vi "NBreset.vi"(4 "Controller Device Description":string="DLP-IO20") -> ()   [LabVIEW 2013]
uses:
  Global 1.vi
panel:
  out "OK":bool
  out "Ping result":u8 format="%x"
  out "Status":i32=1
  out "Bytes Written 6":i32=5
  out "Bytes Read 6":i32
  out "Read Array 6":i32[](array[numeric])
  out "Write Array 6":i32[](array[numeric])=[5, 53, 6, 0, 0]
  out "Bytes Written 7":i32=5
  out "Bytes Read 7":i32
  out "Read Array 7":i32[](array[numeric])
  out "Write Array 7":i32[](array[numeric])=[5, 53, 7, 0, 0]
  out "Handle":u32=263961288
  # "Netburner Reset Panel"
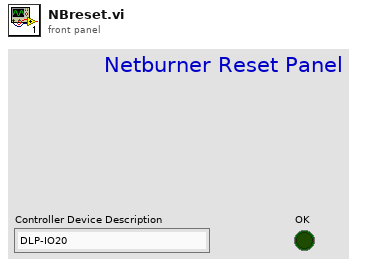
[diagram p1: front panel]
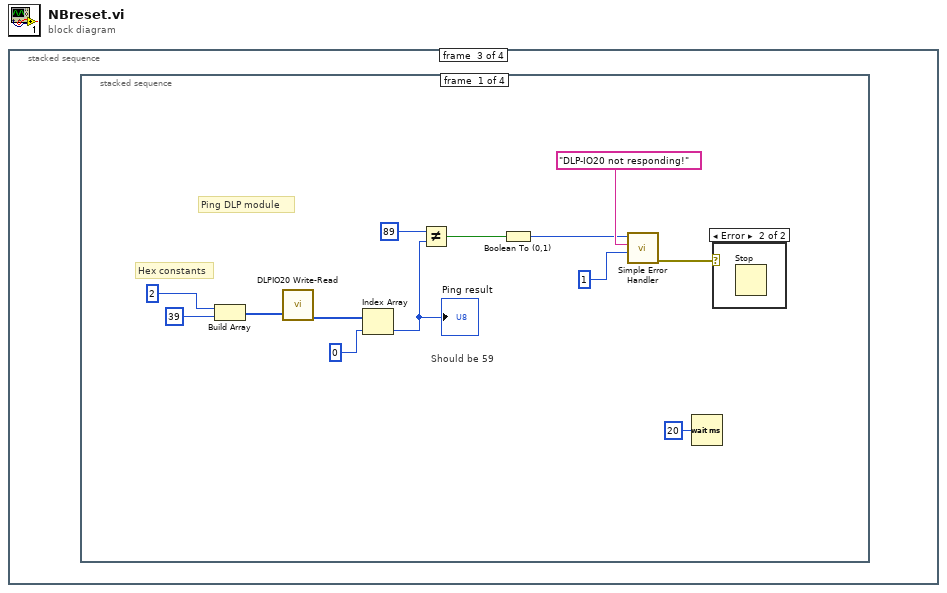
[diagram p0: block diagram]
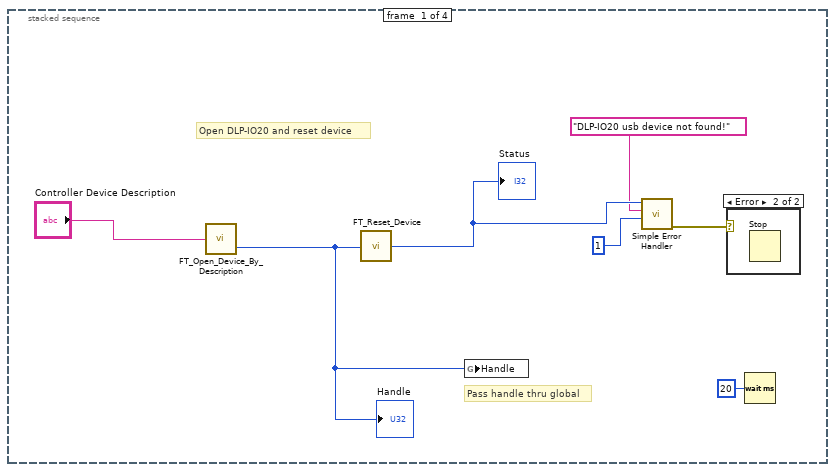
[diagram p2: hidden frame]
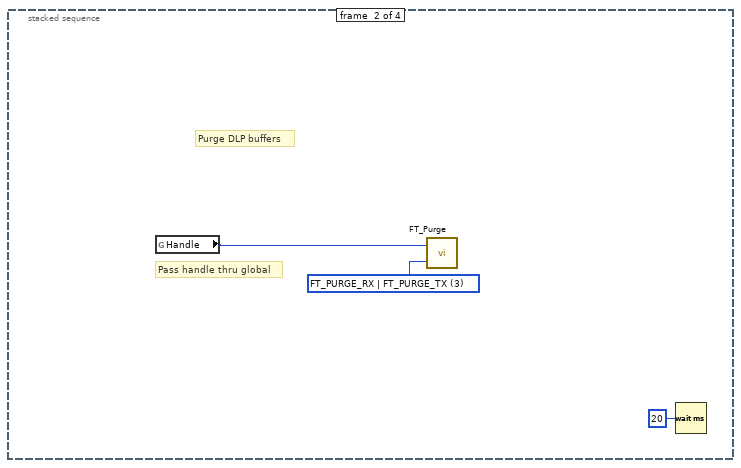
[diagram p4: hidden frame]
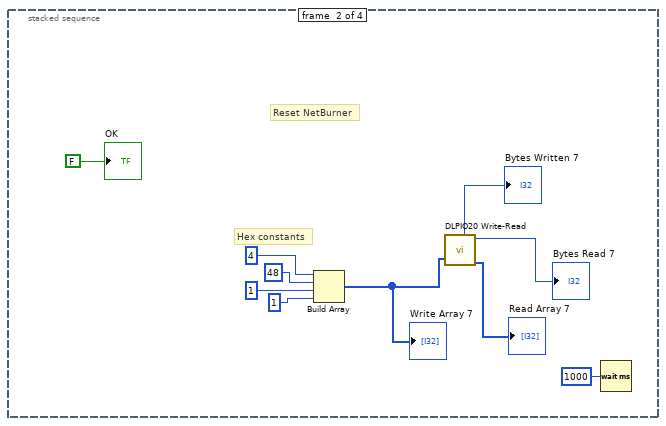
[diagram p6: hidden frame]
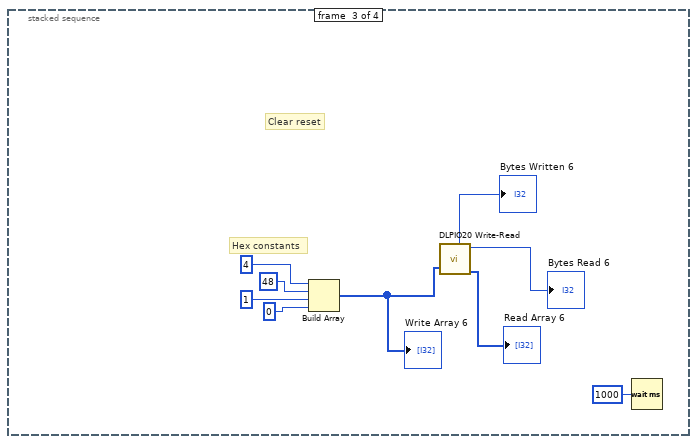
[diagram p7: hidden frame]
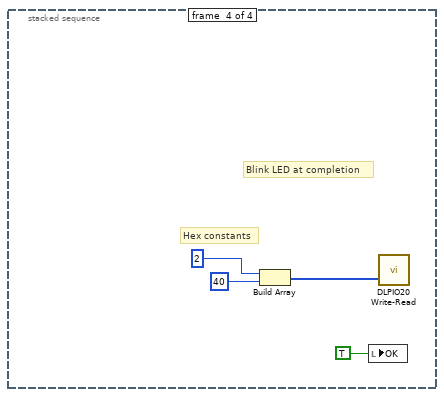
[diagram p8: hidden frame]
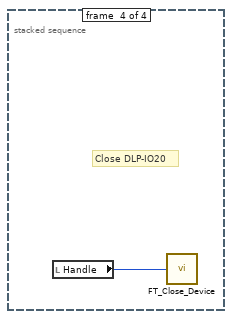
[diagram p9: hidden frame]
diagram:
  n1 = stacked-sequence {
    frame #0 {
      # "Pass handle thru global"
      # "Open DLP-IO20 and reset device"
      n2 = call "FT_Open_Device_By_Description.vi"("Device Description"="Controller Device Description") -> ("Handle"=w5:u32)  [unwired: 1 out]
      "Handle" <- w5
      n3 = call "FT_Reset_Device.vi"("Handle"=w5) -> ("FT_Status"=w4:u32)
      "Status" <- w4
      n4 = global write "Global 1.vi" "Handle"(w5) -> ()
      n5 = call <vilib>:"Simple Error Handler.vi"("error code (no error:0)"=w4, "error source (\" \")"="DLP-IO20 usb device not found!", "type of dialog (OK msg:1)"=1) -> ("error out"=w1:errorcluster)  [unwired: 2 in, 4 out]
      n6 = case shown="Error" w1 {
        frame No Error {
        }
        frame Error {
          n7 = Stop() -> ()  [unwired: 1 in]
        }
      }
      n8 = Wait (ms)(milliseconds to wait=u32 20) -> ()  [unwired: 1 out]
    }
    frame #1 {
      w10 = u32 3 items=["FT_PURGE_RX"=1, "FT_PURGE_TX"=2, "FT_PURGE_RX | FT_PURGE_TX"=3] ("Purge Flags")
      # "Purge DLP buffers"
      # "Pass handle thru global"
      n9 = global read "Global 1.vi" "Handle"() -> (w9:u32)
      n10 = call "FT_Purge.vi"("Purge Flags"=w10, "Handle"=w9) -> ()  [unwired: 1 out]
      n11 = Wait (ms)(milliseconds to wait=u32 20) -> ()  [unwired: 1 out]
    }
    frame #2 {
      n12 = stacked-sequence {
        frame #0 {
          # "Should be 59"
          # "Ping DLP module"
          # "Hex constants"
          n13 = Build Array "Build Array"(u8 2, u8 39) -> (w21:u8[])
          n14 = call "DLPIO20 Write-Read.vi"("Write Buffer"=w21) -> ("Read Buffer Out"=w20:u8[])  [unwired: 3 in, 2 out]
          n15 = Index Array(array=w20, index=u8 0) -> (element=w17:u8)
          "Ping result" <- w17
          n16 = Not Equal?(x=u8 89, y=w17) -> (x != y?=w13:bool)
          n17 = Boolean To (0,1)(Boolean=w13) -> (0, 1=w12:i16)
          n18 = call <vilib>:"Simple Error Handler.vi"("error code (no error:0)"=w12, "error source (\" \")"="DLP-IO20 not responding!", "type of dialog (OK msg:1)"=1) -> ("error out"=w14:errorcluster)  [unwired: 2 in, 4 out]
          n19 = Wait (ms)(milliseconds to wait=u32 20) -> ()  [unwired: 1 out]
          n20 = case shown="Error" w14 {
            frame No Error {
            }
            frame Error {
              n21 = Stop() -> ()  [unwired: 1 in]
            }
          }
        }
        frame #1 {
          # "Reset NetBurner"
          # "Hex constants"
          n22 = Build Array "Build Array"(u8 4, u8 48, u8 1, u8 1) -> (w28:u8[])
          "Write Array 7" <- w28
          n23 = call "DLPIO20 Write-Read.vi"("Write Buffer"=w28) -> ("Read Buffer Out"=→"Read Array 7":u8[], "Bytes Read"=→"Bytes Read 7":u32, "Bytes Written"=→"Bytes Written 7":u32)  [unwired: 3 in]
          n24 = Wait (ms)(milliseconds to wait=u32 1000) -> ()  [unwired: 1 out]
          "OK" <- FALSE
        }
        frame #2 {
          # "Clear reset"
          # "Hex constants"
          n25 = Build Array "Build Array"(u8 4, u8 48, u8 1, u8 0) -> (w37:u8[])
          "Write Array 6" <- w37
          n26 = call "DLPIO20 Write-Read.vi"("Write Buffer"=w37) -> ("Read Buffer Out"=→"Read Array 6":u8[], "Bytes Read"=→"Bytes Read 6":u32, "Bytes Written"=→"Bytes Written 6":u32)  [unwired: 3 in]
          n27 = Wait (ms)(milliseconds to wait=u32 1000) -> ()  [unwired: 1 out]
        }
        frame #3 {
          # "Blink LED at completion"
          # "Hex constants"
          n28 = Build Array "Build Array"(u8 2, u8 40) -> (w44:u8[])
          n29 = local write "OK"(TRUE) -> ()
          n30 = call "DLPIO20 Write-Read.vi"("Write Buffer"=w44) -> ()  [unwired: 3 in, 3 out]
        }
      }
    }
    frame #3 {
      # "Close DLP-IO20"
      n31 = local read "Handle"() -> (w47:u32)
      n32 = call "FT_Close_Device.vi"("Handle"=w47) -> ()  [unwired: 1 out]
    }
  }
